vi "Pixel_Scan_Engine_V3.vi"(0 "Pixel Scan Parameters In":T2={"Scan Start Pixel"=1, "Scan End Pixel"=1, "Pixel Start Value (-1 to 1)"=-0.5, "Pixel End Value (-1 to 1)"=0.5, "Number of Steps"=0.1}, 2 "Action":T3(ring), 7 "Initial Mirror Modes":T1, 11 "Initial Pixel Values (-1 to 1)":dbl[](array[numeric]), 13 "Base Save Path":path=path "Not A Path", 14 "Save Data":bool) -> ()   [LabVIEW 2016]
uses:
  Controls/Pixel Scan Parameters.ctl
  Controls/MirrorModes.ctl
  Controls/Standard_Counter_Action.ctl
  Hardware Configuration/Hardware Configuration Controls/Standard Action.ctl
  Controls/StandardAction.ctl
  <vilib>/Utility/file.llb/Write Delimited Spreadsheet (DBL).vi
panel:
  in  "Pixel Scan":bool=TRUE
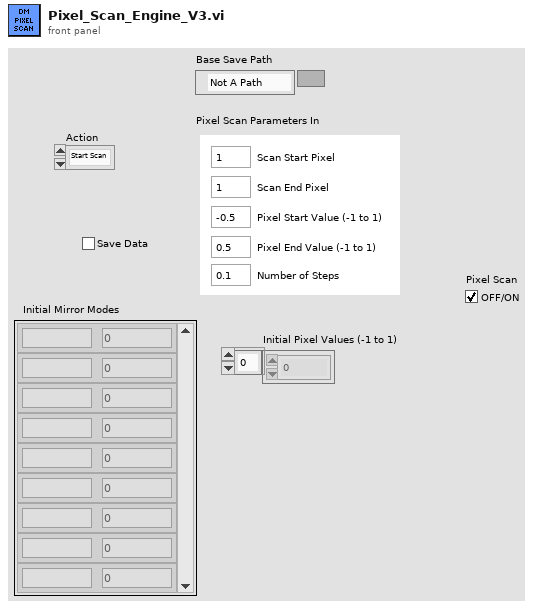
[diagram p1: front panel]
types:
  T1 = typedef "MirrorModes.ctl" = cluster{"Mode":string, "Amplitude":dbl}[]
  T2 = typedef "Pixel Scan Parameters.ctl" = cluster{"Scan Start Pixel":i32, "Scan End Pixel":i32, "Pixel Start Value (-1 to 1)":dbl, "Pixel End Value (-1 to 1)":dbl, "Number of Steps":dbl}
  T3 = enum16{"Start Scan", "Reset Counter", "Write DM", "Get Image", "Update Count", "Exit"}
  T4 = typedef "Standard_Counter_Action.ctl" = enum16{"Initialize", "Update Count", "Get Count"}
  T5 = typedef "Standard Action.ctl" = enum16{"Read", "Write"}
  T6 = typedef "StandardAction.ctl" = enum16{"Read", "Write"}
  T7 = typedef "Camera Parameters.ctl" = cluster{"Edge Filter":string, "Pixel Clock":i32, "Frame Rate":dbl, "Exposure Time (ms)":dbl, "Black Level Offset":i32, "Master Gain":i32, "Master Gain Bool":bool, "Hot Pixel Correction":bool, "Frames Per Capture":u32, "Frame Accumulations":u32}
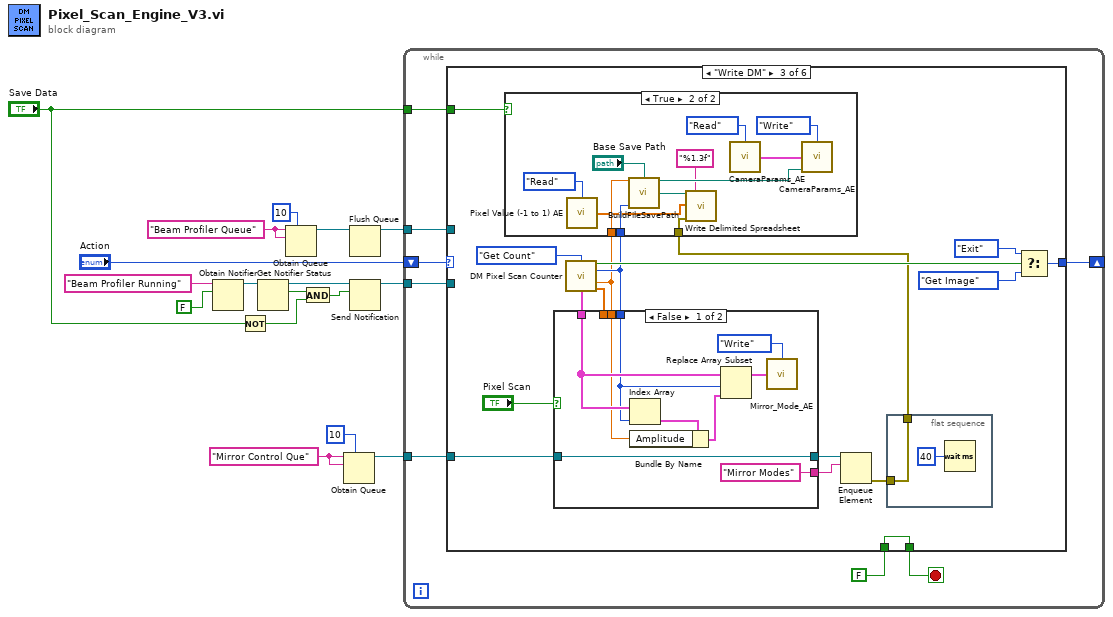
[diagram p0: block diagram]
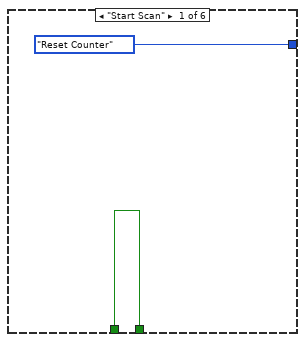
[diagram p2: hidden frame]
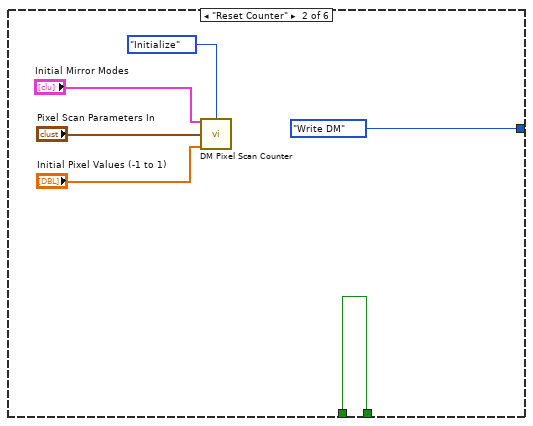
[diagram p3: hidden frame]
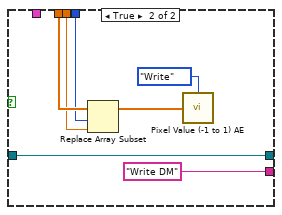
[diagram p4: hidden frame]
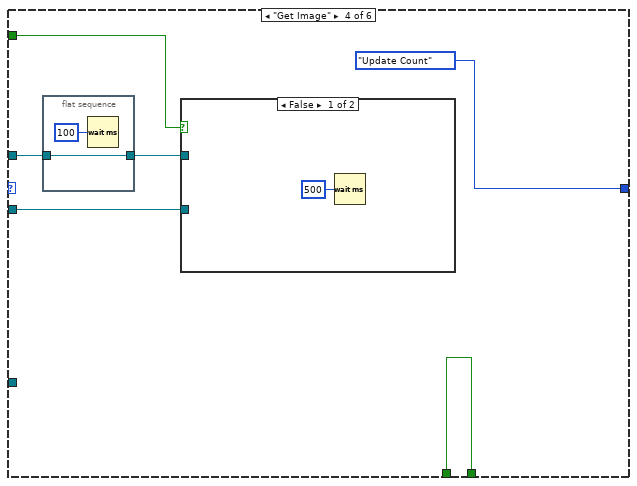
[diagram p6: hidden frame]
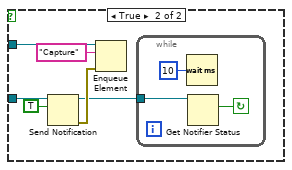
[diagram p7: hidden frame]
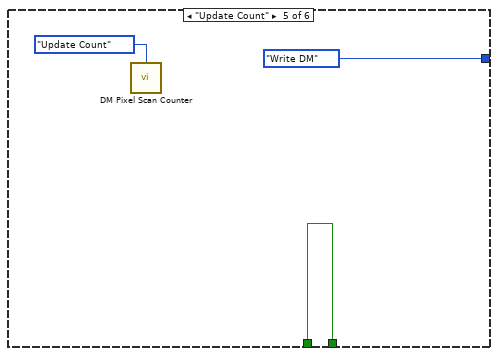
[diagram p8: hidden frame]
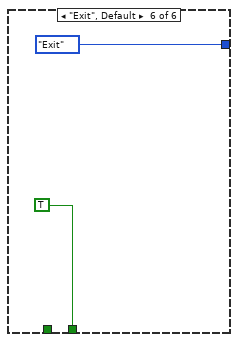
[diagram p9: hidden frame]
diagram:
  w3 = "Mirror Control Que" ("name (unnamed)")
  w14 = "Beam Profiler Queue" ("name (unnamed)")
  n1 = Obtain Notifier(name (unnamed)="Beam Profiler Running", notification data type=FALSE) -> (notifier out=w9:refnum<notifier>)  [unwired: 2 in, 2 out]
  n2 = Not(x="Save Data") -> (.not. x?=w4:bool)
  n3 = Get Notifier Status(notifier=w9) -> (notifier out=w8:refnum<notifier>, current notification=w7:bool)  [unwired: 1 in, 3 out]
  n4 = Obtain Queue(max queue size (-1, unlimited)=10, name (unnamed)=w14, element data type=w14) -> (queue out=w12:refnum<queue>)  [unwired: 2 in, 2 out]
  n5 = And(x=w7, y=w4) -> (x .and. y?=w6:bool)
  n6 = Obtain Queue(max queue size (-1, unlimited)=10, name (unnamed)=w3, element data type=w3) -> (queue out=w1:refnum<queue>)  [unwired: 2 in, 2 out]
  n7 = Flush Queue(queue=w12) -> (queue out=w11:refnum<queue>)  [unwired: 1 in, 2 out]
  n8 = Send Notification(notification=w6, notifier=w8) -> (notifier out=w10:refnum<notifier>)  [unwired: 1 in, 1 out]
  n9 = while {
    shift-right: [w22] -> _
    shift-left: "Action" -> [w25]
    tunnel: w11 -> [w21]
    tunnel: w10 -> [w20]
    tunnel: "Save Data" -> [w19]
    tunnel: w1 -> [w18]
    stop <- w24 stop-if-true
    n10 = case shown="\"Write DM\"" w25 {
      tunnel: [w27 w30 w45 w86 w100 TRUE] -> w24
      tunnel: FALSE -> [w27 w30 w45 w86 w100 _]
      tunnel: [T3."Reset Counter" ("Action") T3."Write DM" ("Action") w46 T3."Update Count" ("Action") T3."Write DM" ("Action") T3."Exit" ("Action")] -> w22
      tunnel: w21 -> [_ _ _ w82 _ _]
      tunnel: w20 -> [_ _ _ w84 _ _]
      tunnel: w19 -> [_ _ w41 w83 _ _]
      tunnel: w18 -> [_ _ w40 _ _ _]
      frame "Start Scan" {
      }
      frame "Reset Counter" {
        n11 = call "DM Pixel Scan Counter.vi"("Initial Mirror Modes"="Initial Mirror Modes", "Action"=Standard_Counter_Action."Initialize", "Pixel Scan Parameters In"="Pixel Scan Parameters In", "Initial Pixel Values (-1 to 1)"="Initial Pixel Values (-1 to 1)") -> ()  [unwired: 7 in, 5 out]
      }
      frame "Write DM" {
        n12 = call "DM Pixel Scan Counter.vi"("Action"=Standard_Counter_Action."Get Count") -> ("Scan Done"=w47:bool, "DM Pixel"=w43:i32, "Normalized DM Pixel Value"=w42:dbl, "Initial Mirror Modes OUT"=w39:T1, "Initial Pixel Values OUT"=w48:dbl[])  [unwired: 10 in]
        n13 = case shown="True" w41 {
          tunnel: w43 -> [_ w77]
          tunnel: w42 -> [_ w76]
          tunnel: w34 -> [_ w69]
          frame False {
          }
          frame True {
            n14 = call "Pixel Value (-1 to 1) AE.vi"("Action"=Standard_Action."Read") -> ("Pixel Value (-1 to 1) Out"=w70:dbl[])  [unwired: 14 in]
            n15 = call "BuildFileSavePath.vi"("Pixel Value"=w76, "Base Path"="Base Save Path", "DM Pixel"=w77) -> ("DBL File Path"=w75:path, "TXT File Path"=w74:path)  [unwired: 11 in]
            n16 = call-poly <vilib>:"Write Delimited Spreadsheet.vi"("file path (dialog if empty)"=w74, "format (%.3f)"="%1.3f" ("format string"), "1D data"=w70, "error in (no error)"=w69) -> ()  [unwired: 10 in, 2 out]
            n17 = call "CameraParams_AE.vi"("Action"=StandardAction."Read") -> ("Camera Parameters Out"=w80:T7)  [unwired: 13 in, 1 out]
            n18 = call "CameraParams_AE.vi"("Action"=StandardAction."Write", "Camera Parameters"=w80, "Save Path"=w75) -> ()  [unwired: 11 in, 2 out]
          }
        }
        n19 = case shown="False" "Pixel Scan" {
          tunnel: w48 -> [_ w68]
          tunnel: w43 -> [w53 w67]
          tunnel: w42 -> [w56 w66]
          tunnel: w40 -> [w55 w64]
          tunnel: w39 -> [w57 _]
          tunnel: [w55 w64] -> w38
          tunnel: ["Mirror Modes" ("name (unnamed)") "Write DM" ("name (unnamed)")] -> w37
          frame False {
            n20 = Index Array(array=w57, index=w53) -> (element=w60:cluster{"Mode":string, "Amplitude":dbl})
            n21 = Bundle By Name(cluster=w60, "Amplitude"=w56) -> (w61:cluster{"Mode":string, "Amplitude":dbl})
            n22 = Replace Array Subset(array=w57, new element=w61, index=w53) -> (w59:T1)
            n23 = call "Mirror_Mode_AE.vi"("Action"=Standard_Action."Write", "Mirror Modes In"=w59) -> ()  [unwired: 13 in, 1 out]
          }
          frame True {
            n24 = Replace Array Subset(array=w68, new element=w66, index=w67) -> (w65:dbl[])
            n25 = call "Pixel Value (-1 to 1) AE.vi"("Action"=Standard_Action."Write", "Pixel Value (-1 to 1)"=w65) -> ()  [unwired: 13 in, 1 out]
          }
        }
        n26 = Enqueue Element(queue=w38, element=w37) -> (error out=w35:errorcluster)  [unwired: 2 in, 2 out]
        n27 = flat-sequence {
          tunnel: w35 -> [w52]
          tunnel: [w52] -> w34
          frame #0 {
            n28 = Wait (ms)(milliseconds to wait=u32 40) -> ()  [unwired: 1 out]
          }
        }
        n29 = Select(t=T3."Exit" ("Action"), s=w47, f=T3."Get Image" ("Action")) -> (s? t:f=w46:T3)
      }
      frame "Get Image" {
        n30 = flat-sequence {
          tunnel: [w88] -> w81
          tunnel: w82 -> [w88]
          frame #0 {
            n31 = Wait (ms)(milliseconds to wait=u32 100) -> ()  [unwired: 1 out]
          }
        }
        n32 = case shown="False" w83 {
          tunnel: w84 -> [_ w95]
          tunnel: w81 -> [_ w94]
          frame False {
            n33 = Wait (ms)(milliseconds to wait=u32 500) -> ()  [unwired: 1 out]
          }
          frame True {
            n34 = Send Notification(notification=TRUE, notifier=w95) -> (notifier out=w90:refnum<notifier>, error out=w93:errorcluster)  [unwired: 1 in]
            n35 = Enqueue Element(queue=w94, element="Capture", error in (no error)=w93) -> ()  [unwired: 1 in, 3 out]
            n36 = while {
              tunnel: w90 -> [w98]
              stop <- w96 continue-if-true
              n37 = Wait (ms)(milliseconds to wait=u32 10) -> ()  [unwired: 1 out]
              n38 = Get Notifier Status(notifier=w98) -> (current notification=w96:bool)  [unwired: 1 in, 4 out]
            }
          }
        }
      }
      frame "Update Count" {
        n39 = call "DM Pixel Scan Counter.vi"("Action"=Standard_Counter_Action."Update Count") -> ()  [unwired: 10 in, 5 out]
      }
      frame "Exit", Default {
      }
    }
  }
